vi "pathfinder generate.vi"(8 "error in":errorcluster, 11 "trajectory length":i32) -> (0 "error out":errorcluster, 3 "Segments":T1[](array[typedef]))   [LabVIEW 2018, in "Pathfinder.lvlib"]
doc: "CAPI int pathfinder_generate_LabVIEW(Segment *segments);"
uses:
  Pathfinder.lvlib
  Segment.ctl
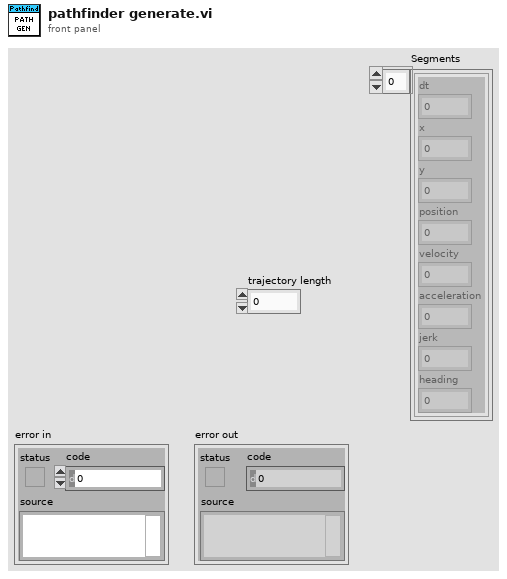
[diagram p1: front panel]
types:
  T1 = typedef "Pathfinder.lvlib/Segment.ctl" = cluster{"dt":dbl, "x":dbl, "y":dbl, "position":dbl, "velocity":dbl, "acceleration":dbl, "jerk":dbl, "heading":dbl}
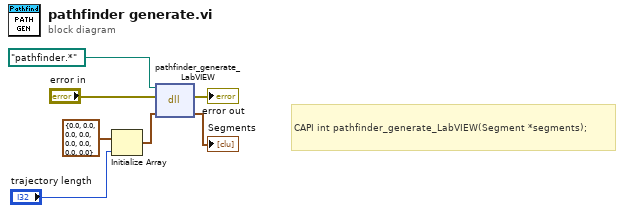
[diagram p0: block diagram]
diagram:
  # "CAPI int pathfinder_generate_LabVIEW(Segment *segments);"
  n1 = Initialize Array(T1 {"dt"=0.0, "x"=0.0, "y"=0.0, "position"=0.0, "velocity"=0.0, "acceleration"=0.0, "jerk"=0.0, "heading"=0.0} ("segment"), "trajectory length") -> (w4:T1[])
  n2 = dll-call lib="?" fn="pathfinder_generate_LabVIEW"(path in=path "pathfinder.*", error in="error in", "segments"=w4) -> (error out=→"error out":errorcluster, "segments"=→"Segments":T1[])  [unwired: 2 in, 1 out]
